vi "Init Communication.vi"(8 "error in (no error)":errorcluster, 10 "VISA resource name":refnum<visa-resource-name>, 11 "Serial Communication in":refnum<class "Serial Communication.lvclass">) -> (0 "error out":errorcluster, 3 "Serial Communication out":refnum<class "Serial Communication.lvclass">)   [LabVIEW 2018, in "Serial Communication.lvclass"]
uses:
  Serial Communication.lvclass
  Serial Communication.lvclass/Serial Communication.ctl
  <vilib>/Instr/_visa.llb/VISA Configure Serial Port (Instr).vi
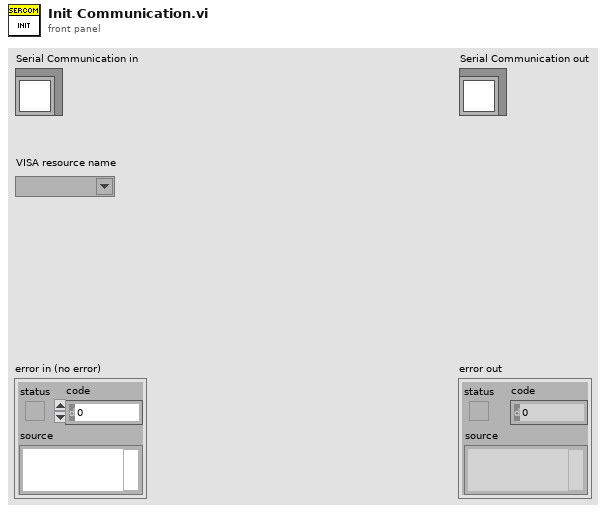
[diagram p1: front panel]
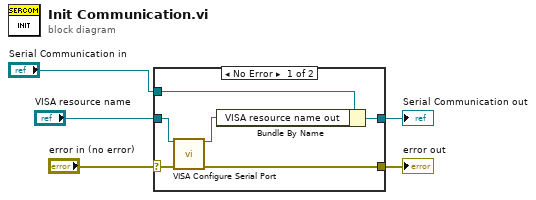
[diagram p0: block diagram]
diagram:
  n1 = case shown="No Error" "error in (no error)" {
    selector: "error in (no error)" -> [w11 w13]
    tunnel: [w10 w13] -> w4
    tunnel: [w8 w12] -> w2
    tunnel: "Serial Communication in" -> [w9 w12]
    tunnel: "VISA resource name" -> [w6 _]
    frame No Error {
      n2 = call-poly "VISA Configure Serial Port"("VISA resource name"=w6, "error in (no error)"=w11) -> ("VISA resource name out"=w7:refnum<visa-resource-name>, "error out"=w10:errorcluster)  [unwired: 12 in]
      n3 = Bundle By Name(cluster=w9, "VISA resource name out"=w7) -> (w8:refnum<class "Serial Communication.lvclass">)
    }
    frame Error {
    }
  }
  "error out" <- w4
  "Serial Communication out" <- w2
